vi "Bus Interface.vi"(0 "AddressSpace":refnum<class "AddressSpace.lvclass">, 1 "abort":bool, 5 "instruction":T2, 9 "input valid":bool) -> (6 "response":T1, 10 "done":bool, 14 "ready for input":bool)   [LabVIEW 2017, in "ThreePhasePLL.lvlib" / "AddressSpace.lvclass"]
uses:
  AddressSpace.lvclass
  <instrlib>/_niInstr/Instruction Framework/v1/FPGA/Interfaces/Address Space/Address Space Instruction.ctl
  <instrlib>/_niInstr/Instruction Framework/v1/FPGA/Typedefs/Response.ctl
  AddressSpace.lvclass/AddressSpace.ctl
  <vilib>/Utility/error.llb/Clear Errors.vi
  <vilib>/rvi/Emulation/niFpgaSctlEmulationGetInTimedLoop.vi
  <vilib>/rvi/Emulation/niFpgaProcessEmulError.vi
  <vilib>/rvi/DataTransferAndStorage/Container/Common/niFpgaContainerGetUniqueNameForEmu.vi
  <vilib>/rvi/Memory/Memory_Emulation/nirvimemoryEmulationManagerCache_SetValue.vi
  <vilib>/rvi/Memory/Memory_Emulation/nirvimemoryEmulationManagerCache_GetValue.vi
  <vilib>/rvi/Memory/Memory_Emulation/nirvimemoryEmulationManagerCache_ReleaseExclusive.vi
  <vilib>/rvi/Memory/Memory_Emulation/nirvimemoryEmulationManagerCache_InsertValue.vi
  <vilib>/rvi/Memory/Memory_Emulation/niFpgaMemoryEmulationValidateCache.vi
  <vilib>/rvi/Memory/Memory_Emulation/nirvimemoryEmulationManagerCache_MakeExclusive.vi
  <vilib>/rvi/Memory/Memory_Emulation/niFpgaMemoryEmulationCacheClearOnFirstRun.vi
  <vilib>/rvi/Emulation/niFpgaEmulationIsFPGAContextNoSignature.vi
  <vilib>/rvi/DataTransferAndStorage/Container/Common/niFpgaContainerExecOnDevCompGetState.vi
  <vilib>/rvi/DataTransferAndStorage/Container/XNode/niFpgaContainer.xnode
  <vilib>/rvi/DataTransferAndStorage/Register/Emulation/niFpgaRegisterEmulationRefIn.vi
  <instrlib>/_niInstr/Instruction Framework/v1/FPGA/Typedefs/niInstr Instruction Framework v1 FPGA.lvlib
  <instrlib>/_niInstr/Instruction Framework/v1/FPGA/Interfaces/Address Space/Address Space.lvclass
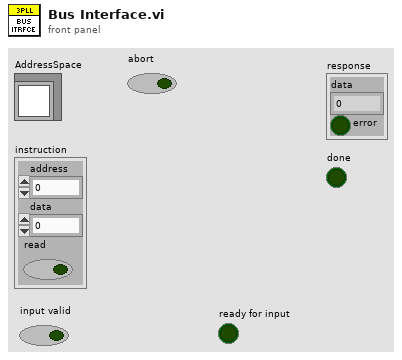
[diagram p1: front panel]
types:
  T1 = typedef "niInstr Instruction Framework v1 FPGA.lvlib/Response.ctl" = cluster{"data":u64, "error":bool}
  T2 = typedef "niInstr Instruction Framework Interfaces v1 FPGA.lvlib/Address Space.lvclass/Address Space Instruction.ctl" = cluster{"address":u32, "data":u64, "read":bool}
  T3 = cluster{"proportional gain":sgl, "integral gain":sgl}
  T4 = cluster{"output high (Inf)":sgl, "output low (-Inf)":sgl}
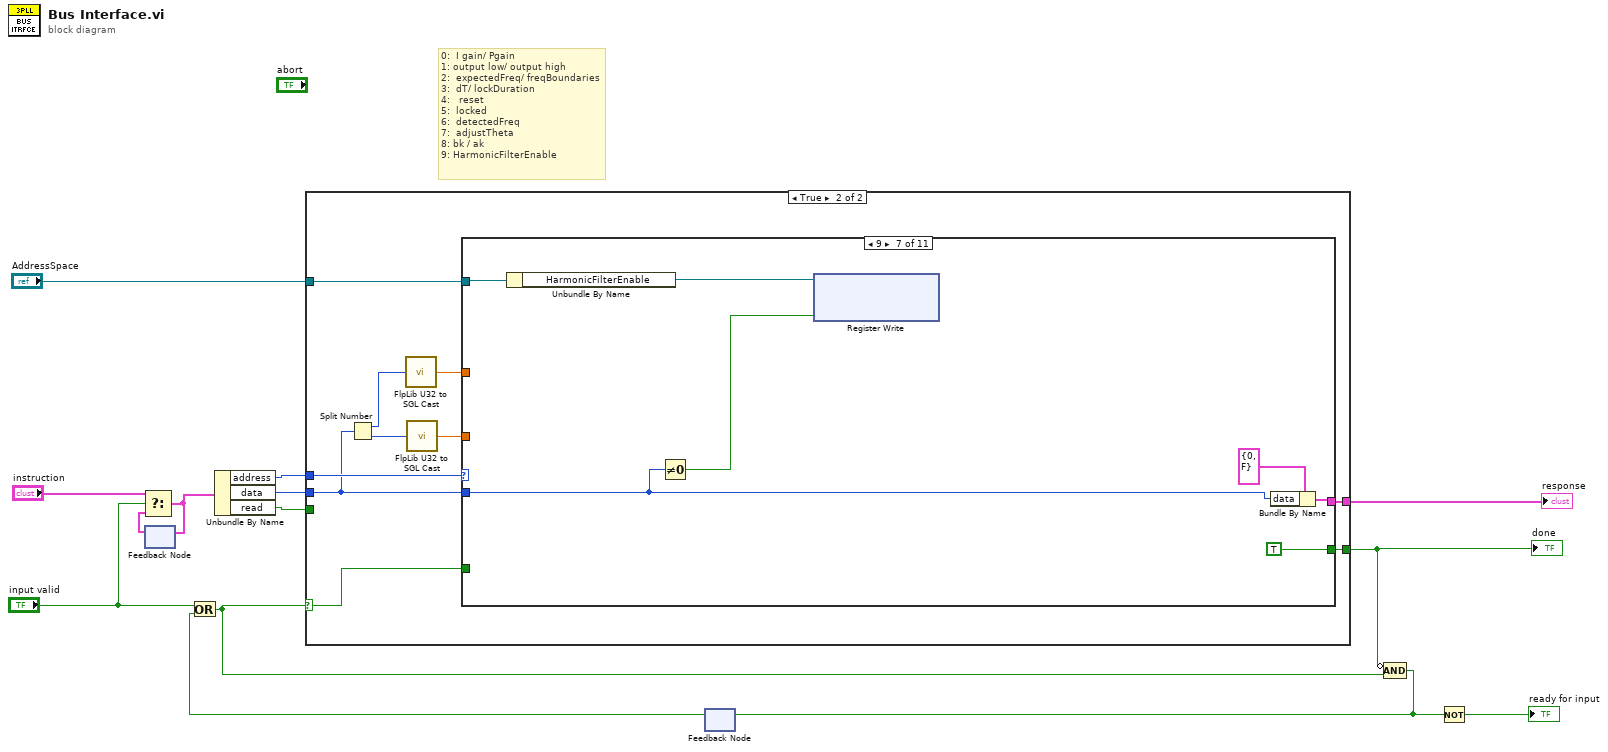
[diagram p0: block diagram]
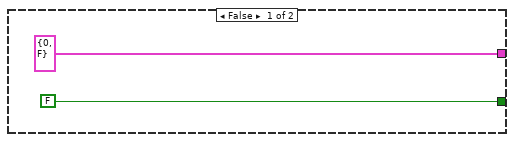
[diagram p2: hidden frame]
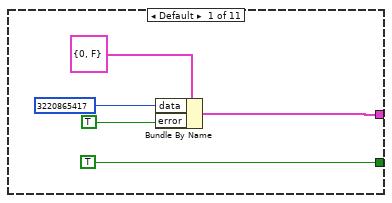
[diagram p3: hidden frame]
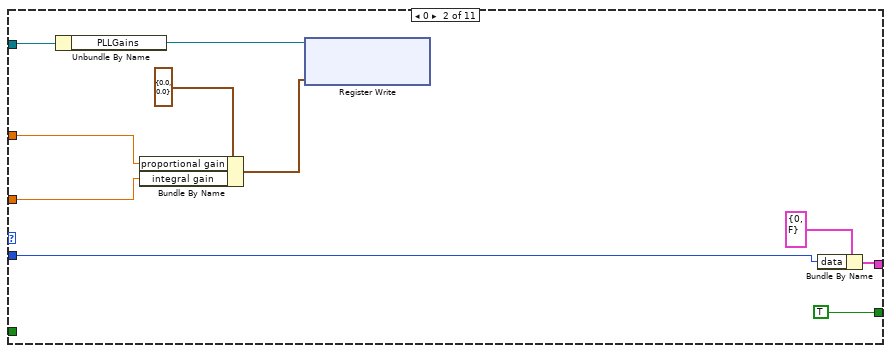
[diagram p4: hidden frame]
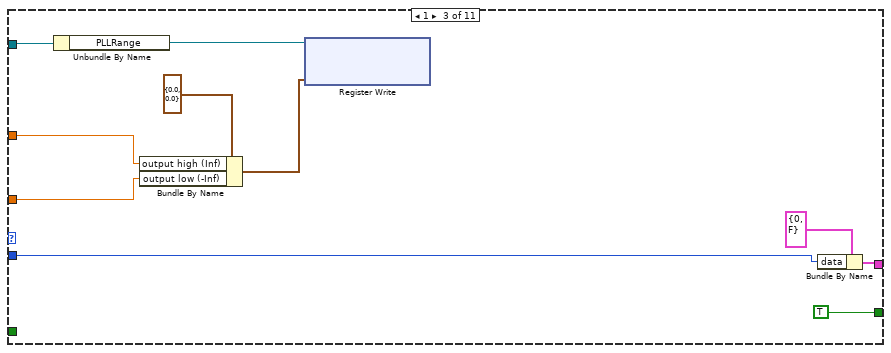
[diagram p5: hidden frame]
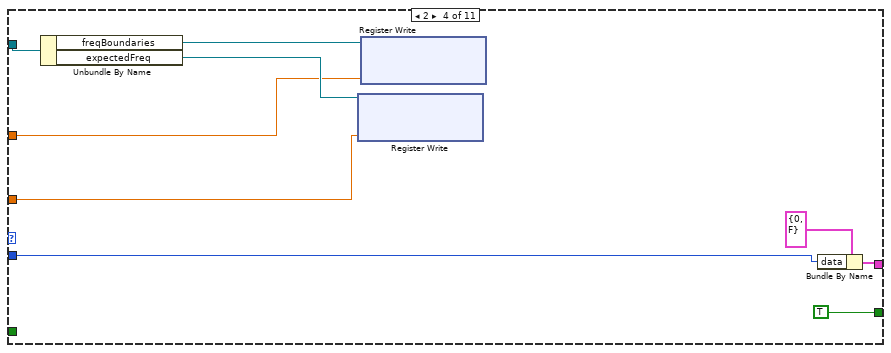
[diagram p6: hidden frame]
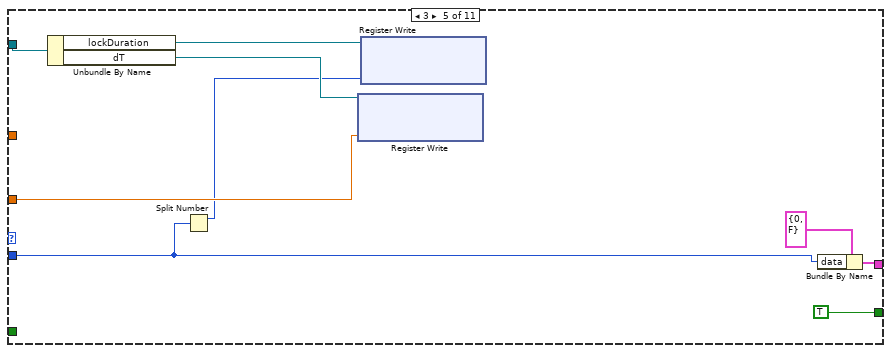
[diagram p7: hidden frame]
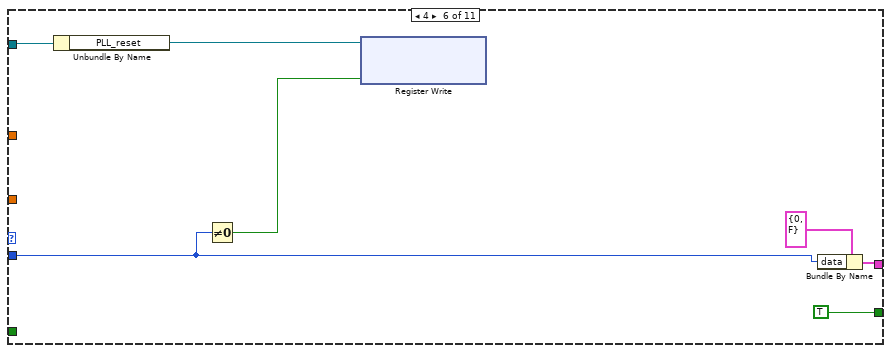
[diagram p8: hidden frame]
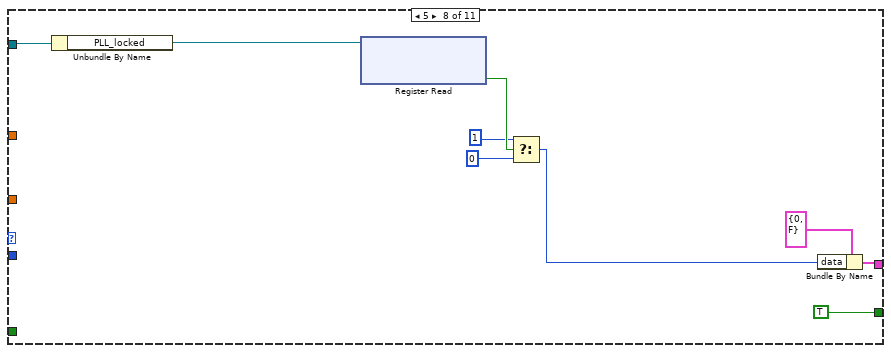
[diagram p9: hidden frame]
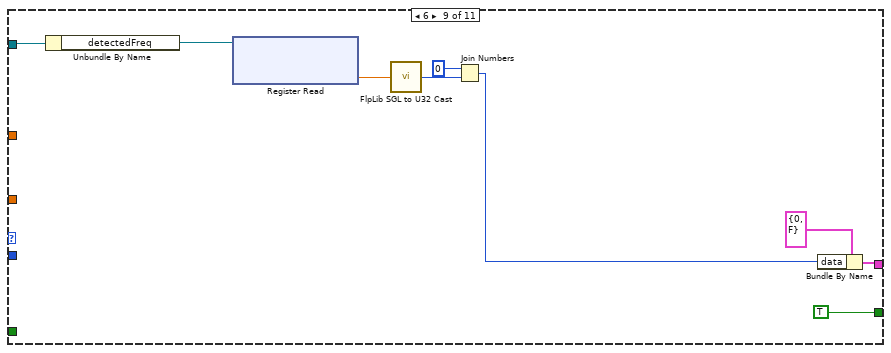
[diagram p10: hidden frame]
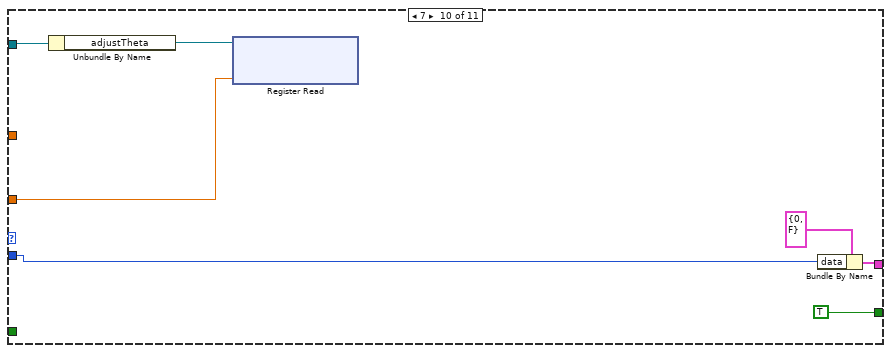
[diagram p11: hidden frame]
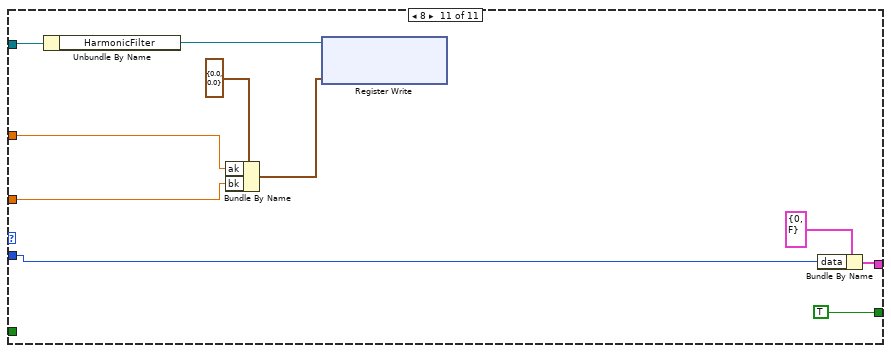
[diagram p12: hidden frame]
diagram:
  # "0:  I gain/ Pgain\n1: output low/ output high\n2:  expectedFreq/ freqBoundaries\n3:  dT/ lockDuration\n4:   reset\n5:  locked\n6:  detectedFreq\n7:  adjustTheta\n8: bk / ak\n9: HarmonicFilterEnable"
  n1 = feedback #1() -> (w14:T2)  [unwired: 1 in]
  n2 = Select(t="instruction", s="input valid", f=w14) -> (s? t:f=w13:T2)
  n3 = feedback-in #1(w13) -> ()
  n4 = Unbundle By Name(w13) -> ("address"=w10:u32, "data"=w11:u64, "read"=w12:bool)
  n5 = feedback #2() -> (w7:bool)  [unwired: 1 in]
  n6 = Or(x="input valid", y=w7) -> (x .or. y?=w8:bool)
  n7 = case shown="True" w8 {
    selector: w8 -> [_ w22]
    tunnel: w12 -> [_ _]
    tunnel: w10 -> [_ w26]
    tunnel: w11 -> [_ w21]
    tunnel: [T1 {"data"=0, "error"=FALSE} ("response") w25] -> w3
    tunnel: [FALSE ("Output Valid") w24] -> w2
    tunnel: "AddressSpace" -> [_ w23]
    frame False {
    }
    frame True {
      n8 = Split Number(x=w21) -> (hi(x)=w18:u32, lo(x)=w20:u32)
      n9 = call <userlib>:"FlpLib U32 to SGL Cast.vi"("x"=w18) -> ("y"=w17:sgl)  [unwired: 4 in]
      n10 = call <userlib>:"FlpLib U32 to SGL Cast.vi"("x"=w20) -> ("y"=w19:sgl)  [unwired: 4 in]
      n11 = case shown="9" w26 {
        tunnel: w21 -> [_ w34 w46 w58 w62 w71 w78 _ _ w103 w113]
        tunnel: [w28 w33 w45 w57 w67 w74 w81 w90 w99 w106 w116] -> w25
        tunnel: [TRUE ("done") TRUE ("done") TRUE ("done") TRUE ("done") TRUE ("done") TRUE ("done") TRUE ("done") TRUE ("done") TRUE ("done") TRUE ("done") TRUE ("done")] -> w24
        tunnel: w23 -> [_ w41 w51 w60 w69 w76 w83 w92 w101 w108 w118]
        tunnel: w22 -> [_ _ _ _ _ _ _ _ _ _ _]
        tunnel: w19 -> [_ w37 w48 w52 w63 _ _ _ _ w102 w110]
        tunnel: w17 -> [_ w38 w49 w53 _ _ _ _ _ _ w111]
        frame Default {
          n12 = Bundle By Name(cluster=T1 {"data"=0, "error"=FALSE} ("response"), "data"=u64 3220865417, "error"=TRUE) -> (w28:T1)
        }
        frame 0 {
          n13 = Unbundle By Name(w41) -> ("PLLGains"=w40:refnum<k21>)
          n14 = Bundle By Name(cluster=T3 {"proportional gain"=0.0, "integral gain"=0.0} ("Data"), "proportional gain"=w38, "integral gain"=w37) -> (w36:T3)
          n15 = xnode "Register Write"("Data"=w36, "Register In"=w40) -> ()  [unwired: 1 out]
          n16 = Bundle By Name(cluster=T1 {"data"=0, "error"=FALSE} ("response"), "data"=w34) -> (w33:T1)
        }
        frame 1 {
          n17 = Unbundle By Name(w51) -> ("PLLRange"=w50:refnum<k21>)
          n18 = Bundle By Name(cluster=T4 {"output high (Inf)"=0.0, "output low (-Inf)"=0.0} ("Data"), "output high (Inf)"=w49, "output low (-Inf)"=w48) -> (w42:T4)
          n19 = xnode "Register Write"("Data"=w42, "Register In"=w50) -> ()  [unwired: 1 out]
          n20 = Bundle By Name(cluster=T1 {"data"=0, "error"=FALSE} ("response"), "data"=w46) -> (w45:T1)
        }
        frame 2 {
          n21 = Unbundle By Name(w60) -> ("freqBoundaries"=w55:refnum<k21>, "expectedFreq"=w54:refnum<k21>)
          n22 = xnode "Register Write"("Data"=w52, "Register In"=w54) -> ()  [unwired: 1 out]
          n23 = xnode "Register Write"("Data"=w53, "Register In"=w55) -> ()  [unwired: 1 out]
          n24 = Bundle By Name(cluster=T1 {"data"=0, "error"=FALSE} ("response"), "data"=w58) -> (w57:T1)
        }
        frame 3 {
          n25 = Unbundle By Name(w69) -> ("lockDuration"=w65:refnum<k21>, "dT"=w64:refnum<k21>)
          n26 = Split Number(x=w62) -> (hi(x)=w61:u32)  [unwired: 1 out]
          n27 = xnode "Register Write"("Data"=w63, "Register In"=w64) -> ()  [unwired: 1 out]
          n28 = xnode "Register Write"("Data"=w61, "Register In"=w65) -> ()  [unwired: 1 out]
          n29 = Bundle By Name(cluster=T1 {"data"=0, "error"=FALSE} ("response"), "data"=w62) -> (w67:T1)
        }
        frame 4 {
          n30 = Unbundle By Name(w76) -> ("PLL_reset"=w72:refnum<k21>)
          n31 = Not Equal To 0?(x=w71) -> (x != 0?=w70:bool)
          n32 = xnode "Register Write"("Data"=w70, "Register In"=w72) -> ()  [unwired: 1 out]
          n33 = Bundle By Name(cluster=T1 {"data"=0, "error"=FALSE} ("response"), "data"=w71) -> (w74:T1)
        }
        frame 9 {
          n34 = Unbundle By Name(w83) -> ("HarmonicFilterEnable"=w79:refnum<k21>)
          n35 = Not Equal To 0?(x=w78) -> (x != 0?=w77:bool)
          n36 = xnode "Register Write"("Data"=w77, "Register In"=w79) -> ()  [unwired: 1 out]
          n37 = Bundle By Name(cluster=T1 {"data"=0, "error"=FALSE} ("response"), "data"=w78) -> (w81:T1)
        }
        frame 5 {
          n38 = Unbundle By Name(w92) -> ("PLL_locked"=w88:refnum<k21>)
          n39 = xnode "Register Read"("Register In"=w88) -> ("Data"=w87:bool)  [unwired: 1 out]
          n40 = Select(t=u64 1 ("data"), s=w87, f=u64 0) -> (s? t:f=w84:u64)
          n41 = Bundle By Name(cluster=T1 {"data"=0, "error"=FALSE} ("response"), "data"=w84) -> (w90:T1)
        }
        frame 6 {
          n42 = Unbundle By Name(w101) -> ("detectedFreq"=w97:refnum<k21>)
          n43 = xnode "Register Read"("Register In"=w97) -> ("Data"=w96:sgl)  [unwired: 1 out]
          n44 = call <userlib>:"FlpLib SGL to U32 Cast.vi"("x"=w96) -> ("y"=w95:u32)  [unwired: 4 in]
          n45 = Join Numbers(hi=u32 0, lo=w95) -> ((hi.lo)=w93:u64)
          n46 = Bundle By Name(cluster=T1 {"data"=0, "error"=FALSE} ("response"), "data"=w93) -> (w99:T1)
        }
        frame 7 {
          n47 = Unbundle By Name(w108) -> ("adjustTheta"=w104:refnum<k21>)
          n48 = xnode "Register Read"("Data"=w102, "Register In"=w104) -> ()  [unwired: 1 out]
          n49 = Bundle By Name(cluster=T1 {"data"=0, "error"=FALSE} ("response"), "data"=w103) -> (w106:T1)
        }
        frame 8 {
          n50 = Unbundle By Name(w118) -> ("HarmonicFilter"=w114:refnum<k21>)
          n51 = Bundle By Name(cluster=cluster{"ak":sgl, "bk":sgl} {"ak"=0.0, "bk"=0.0} ("Data"), "ak"=w111, "bk"=w110) -> (w109:cluster{"ak":sgl, "bk":sgl})
          n52 = xnode "Register Write"("Data"=w109, "Register In"=w114) -> ()  [unwired: 1 out]
          n53 = Bundle By Name(cluster=T1 {"data"=0, "error"=FALSE} ("response"), "data"=w113) -> (w116:T1)
        }
      }
    }
  }
  "done" <- w2
  "response" <- w3
  n54 = Compound Arithmetic op=AND(invert w2, w8) -> (w9:bool)
  n55 = feedback-in #2(w9) -> ()
  n56 = Not(x=w9) -> (.not. x?=→"ready for input":bool)
